vi "IsPDA_SD.vi"   [LabVIEW 2015]
uses:
  DLL/ESLSCDLL.dll
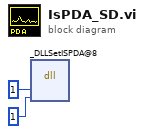
[diagram p0: block diagram]
diagram:
  n1 = dll-call lib="G:/SD/TRANCON/DLL/ESLSCDLL.dll" fn="_DLLSetISPDA@8" ("lwlscdll.dll:DLLSetISPDA")("drv"=u32 1, "set"=u8 1) -> ()  [unwired: 6 in, 2 out]
